vi "Length_15.vi"() -> ()   [LabVIEW 2020]
uses:
  Support/Controls/Cmd_Mouse Popup.ctl
  Support/Controls/Clst_Initialize Input.ctl
  Support/Controls/Clst_Result inspec.ctl
  Support/Controls/Cmd_Var Data IO.ctl
  Variables/Global_Cal Info.vi
panel:
  out "Measured 3":string[][](table) caption="○ 평면도 계산결과 (μm)"
  in  "Measured 2":string[][](table) caption="○ 반복정밀도"
  in  "STD select":string(combo)="1" caption="기준기 Range"
  in  "Spec 변경":bool
  in  "Random":bool
  out "Spec":string[][](table) caption="Spec (명목 직경)"
  out "제목":string
  out "에러 출력":errorcluster
  out "Condition":string[][](table) caption="○ 측정 조건"
  in  "Measured":string[][](table) caption="○ 평면도 측정결과 ( ˝ )"
  out "Load?":bool
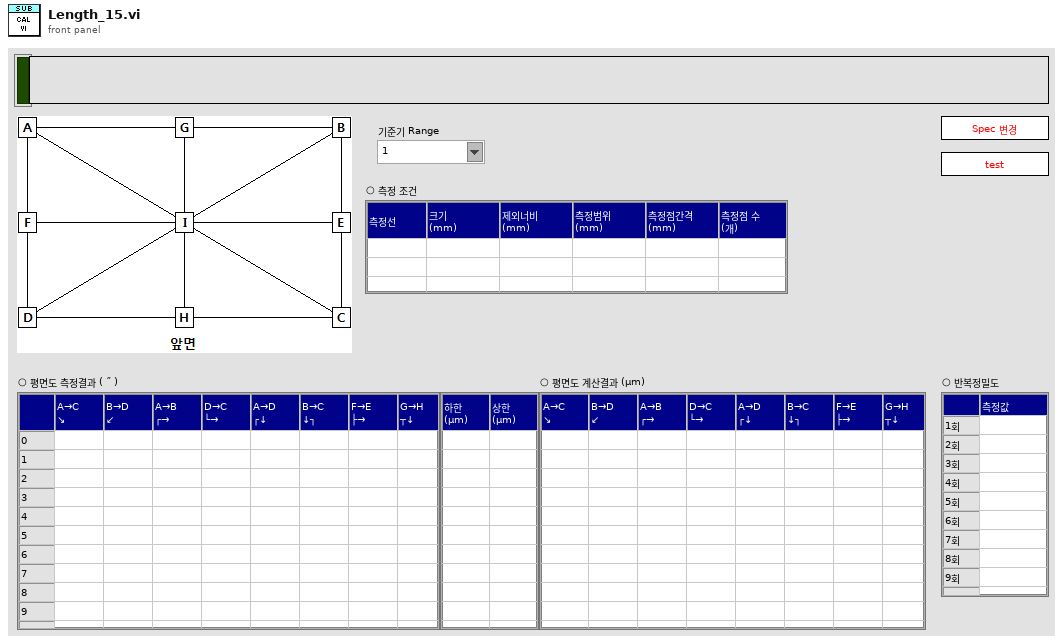
[diagram p1: front panel]
types:
  T1 = typedef "Cmd_Mouse Popup.ctl" = enum16{"활성화", "메뉴선택"}
  T2 = cluster{"Shift":bool, "Ctrl":bool, "Alt":bool, "Cmd":bool, "Opt":bool}
  T3 = typedef "Clst_Initialize Input.ctl" = cluster{"Initialize 1":cluster{"Condition":refnum<vi>[], "Spec":refnum<vi>[], "Measured":refnum<vi>[], "Resolution":refnum<vi>[], "Func_ext":string, "제목":refnum<vi>, "Measured_ADJ":refnum<vi>[]}, "Initialize 2":cluster{"문자열":refnum<vi>[], "콤보박스":refnum<vi>[], "링":refnum<vi>[], "열거형":refnum<vi>[], "테이블":refnum<vi>[], "여러열":refnum<vi>[], "디지털(DBL)":refnum<vi>[], "3D string":refnum<vi>[], "ctrl":refnum<vi>[], "boolean":refnum<vi>[]}}
  T4 = typedef "Clst_Result inspec.ctl" = cluster{"분해능":string, "문자열 1":string, "문자열 2":string, "숫자형 1":i32, "숫자형 2":i32, "숫자형 3":dbl, "문자배열 1D":string[], "문자배열 2D":string[][], "문자배열 3D":string[][][], "문자배열 4D":string[][][][], "불리언 1D":bool[]}
  T5 = typedef "Cmd_Var Data IO.ctl" = enum16{"Condition", "Condition Default", "Condition_Temp", "Resolution", "Resolution Default", "Resolution Old", "Spec", "Spec Default", "Spec Old", "Spec Temp", "Result", "Result2", "Result3", "Result_Temp", "Result_ADJ", "Result_ADJ2", "STD1", "STD2", "STD3", "STD4", "STD5", "STD Temp", "CMC", "CMC Default"}
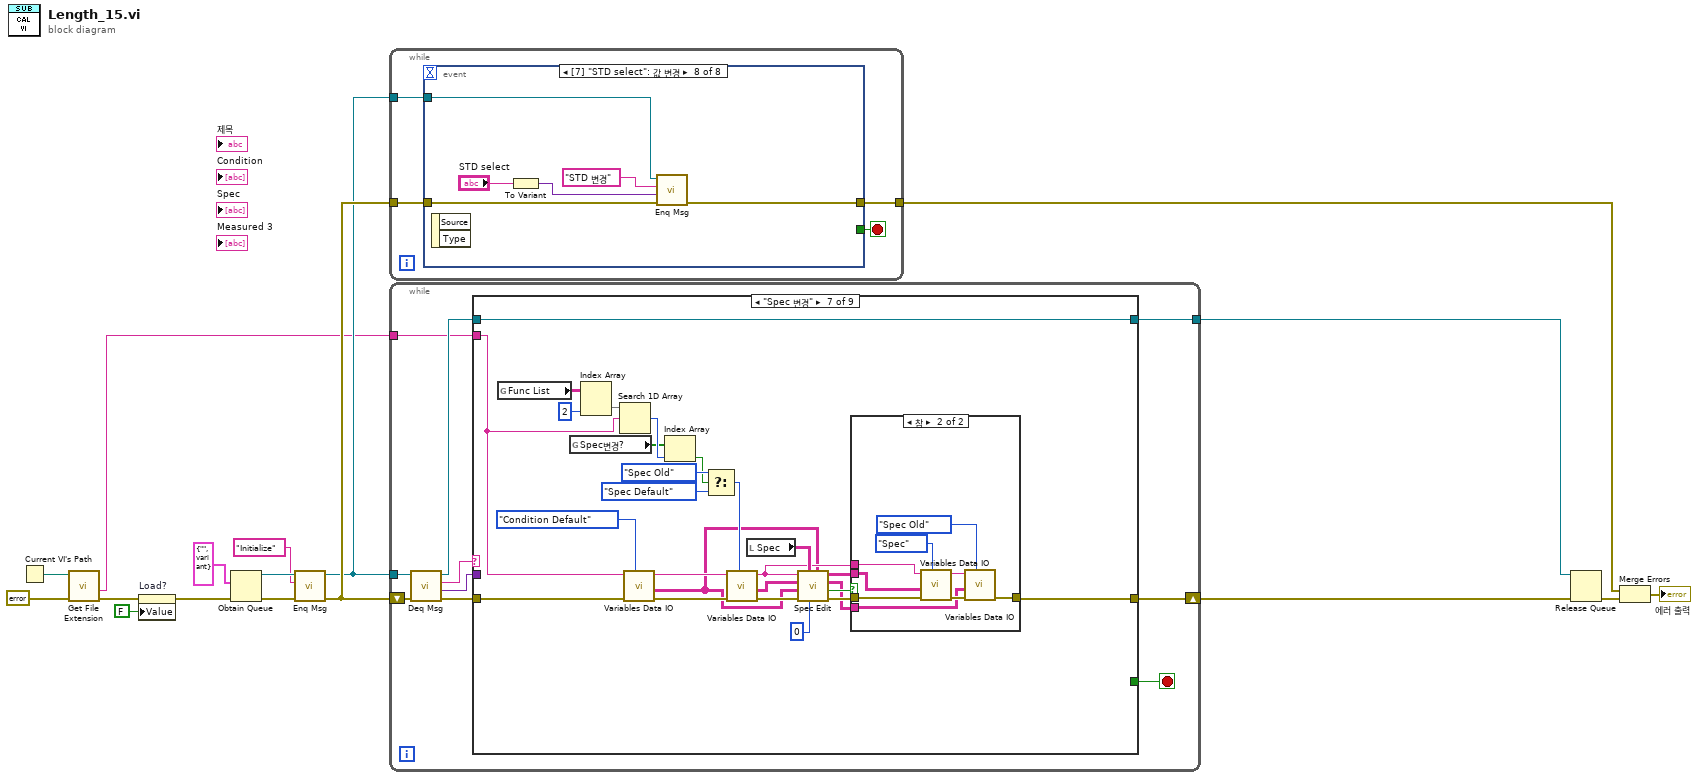
[diagram p0: block diagram]
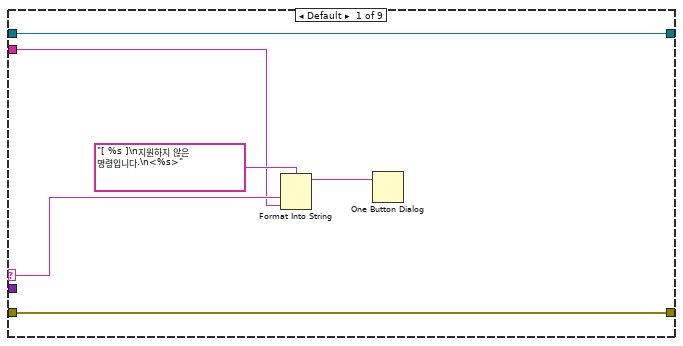
[diagram p2: hidden frame]
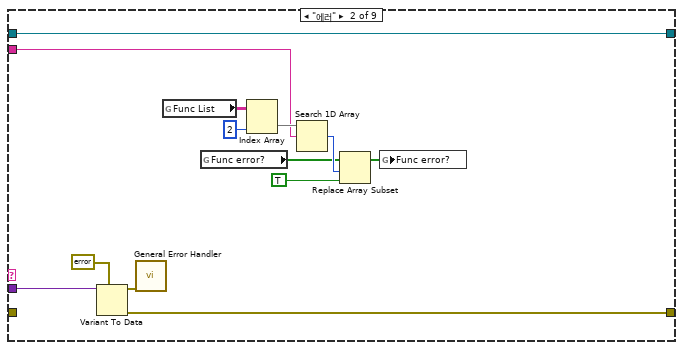
[diagram p3: hidden frame]
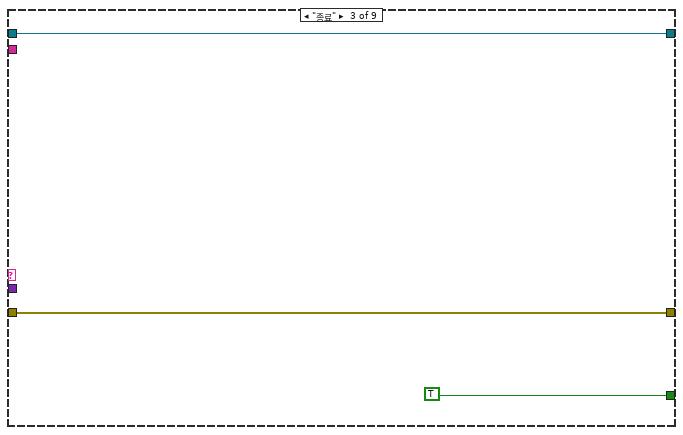
[diagram p4: hidden frame]
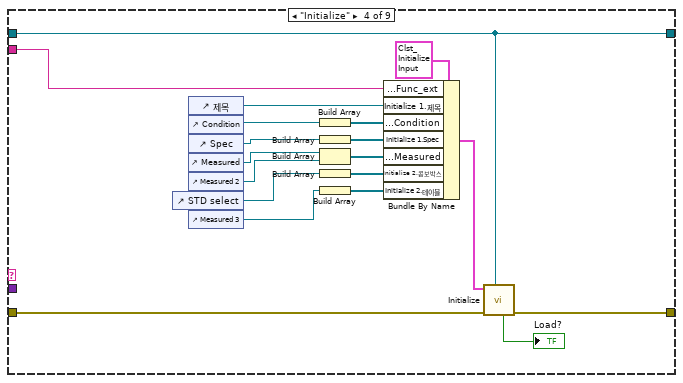
[diagram p5: hidden frame]
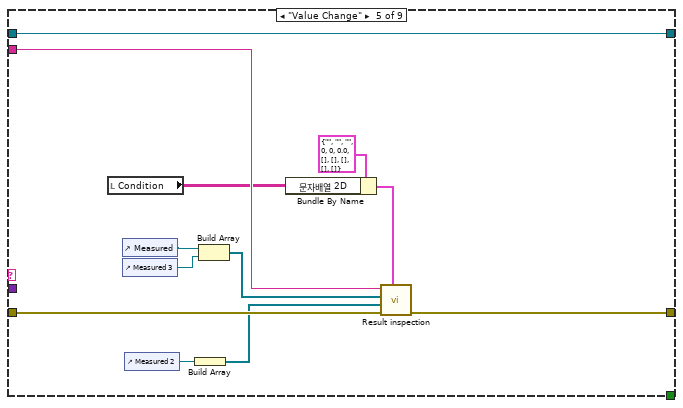
[diagram p6: hidden frame]
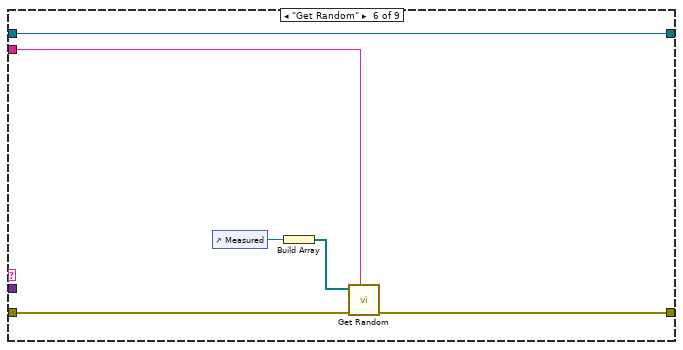
[diagram p7: hidden frame]
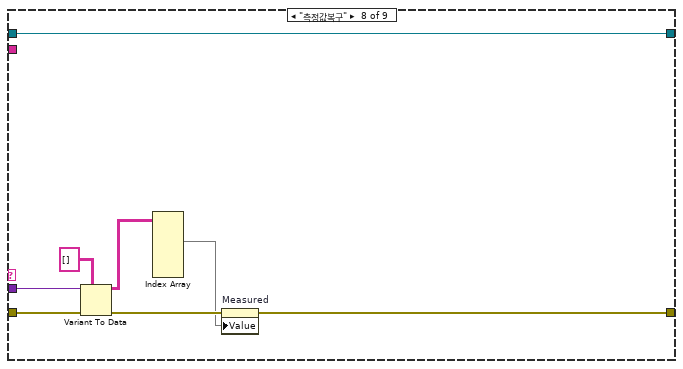
[diagram p9: hidden frame]
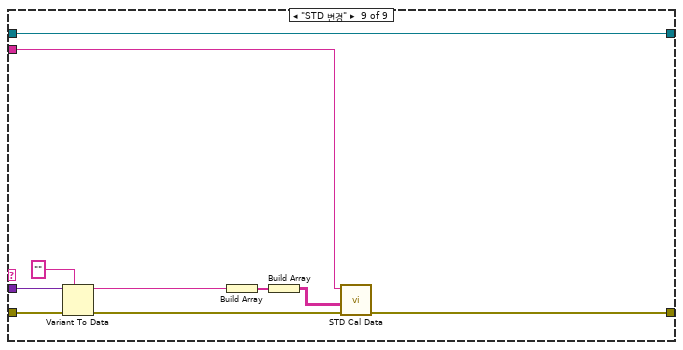
[diagram p10: hidden frame]
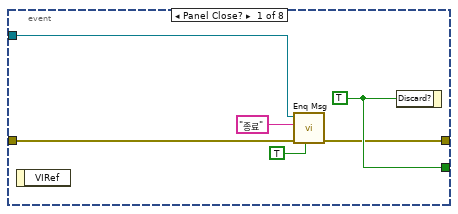
[diagram p11: hidden frame]
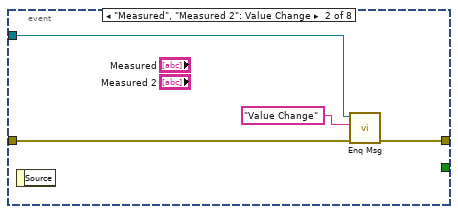
[diagram p12: hidden frame]
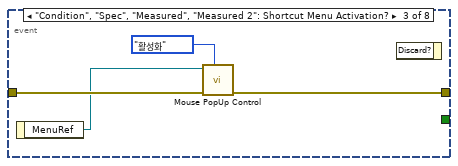
[diagram p13: hidden frame]
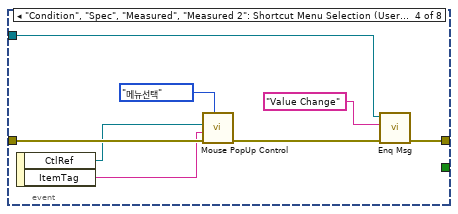
[diagram p14: hidden frame]
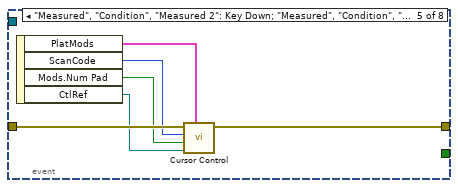
[diagram p15: hidden frame]
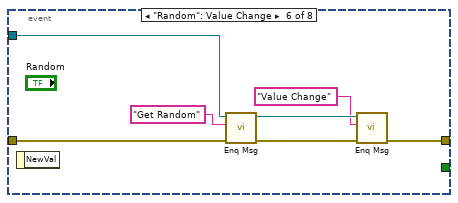
[diagram p16: hidden frame]
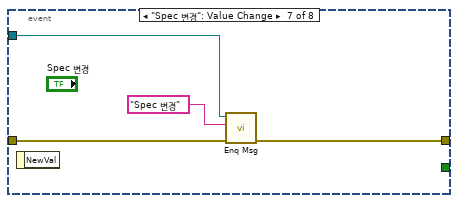
[diagram p17: hidden frame]
diagram:
  n1 = Current VI's Path() -> (path=w5:path)
  n2 = call <vilib>:"Get File Extension.vi"("error in (no error)"=errorcluster {"status"=FALSE, "code"=0, "source"=""} ("에러 상수"), "file"=w5) -> ("error out"=w3:errorcluster, "filename without extension"=w4:string)  [unwired: 5 in, 3 out]
  n3 = property on="Load?" class="Bool (엄격한)"(error in=w3, "Value"=FALSE ("Load?")) -> (error out=w2:errorcluster)  [unwired: 1 in, 1 out]
  n4 = Obtain Queue(element data type=cluster{"메세지":string, "값":variant} {"메세지"="", "값"=variant} ("Message Cluster"), error in (no error)=w2) -> (queue out=w14:refnum<queue>, error out=w16:errorcluster)  [unwired: 3 in, 1 out]
  n5 = call "Enq Msg.vi"("에러 입력(에러 없음)"=w16, "메세지"="Initialize", "큐 입력"=w14) -> ("에러 출력"=w15:errorcluster, "큐 출력"=w12:refnum<queue>)  [unwired: 7 in]
  n6 = while {
    tunnel: w15 -> [w19]
    tunnel: w12 -> [w20]
    tunnel: [w18] -> w9
    stop <- w21 stop-if-true
    n7 = event shown="[7] \"STD select\": 값 변경" {
      selector: _ -> [_ _ _ _ _ _ _ _]
      dyn-events: _ -> [_ _ _ _ _ _ _ _]
      timeout: _ -> [_ _ _ _ _ _ _ _]
      tunnel: [w27 _ _ _ _ _ _ _] -> w21
      tunnel: w20 -> [w25 w31 _ w36 _ w54 w58 w64]
      tunnel: w19 -> [w26 w29 w35 w43 w49 w55 w59 w65]
      tunnel: [w23 w30 w34 w37 w48 w50 w57 w63] -> w18
      event Panel Close? {
        w27 = TRUE ("버림?")
        n8 = event-data() -> ()  [unwired: 1 in, 1 out]
        n9 = call "Enq Msg.vi"("우선순위 메시지?"=TRUE, "에러 입력(에러 없음)"=w26, "메세지"="종료", "큐 입력"=w25) -> ("에러 출력"=w23:errorcluster)  [unwired: 6 in, 1 out]
        n10 = event-data("Discard?"=w27) -> ()  [unwired: 1 in, 1 out]
      }
      event "Measured", "Measured 2": Value Change {
        n11 = event-data() -> ()  [unwired: 1 in, 1 out]
        n12 = call "Enq Msg.vi"("에러 입력(에러 없음)"=w29, "메세지"="Value Change", "큐 입력"=w31) -> ("에러 출력"=w30:errorcluster)  [unwired: 7 in, 1 out]
      }
      event "Condition", "Spec", "Measured", "Measured 2": Shortcut Menu Activation? {
        n13 = event-data() -> ("MenuRef"=w33:refnum<k9>)  [unwired: 1 in]
        n14 = call "Mouse PopUp Control.vi"("type"=Cmd_Mouse_Popup."활성화", "error in"=w35, "메뉴 참조"=w33) -> ("error out"=w34:errorcluster)  [unwired: 8 in]
        n15 = event-data() -> ()  [unwired: 2 in, 1 out]
      }
      event "Condition", "Spec", "Measured", "Measured 2": Shortcut Menu Selection (User) {
        n16 = event-data() -> ("CtlRef"=w41:refnum<vi>, "ItemTag"=w40:string)  [unwired: 1 in]
        n17 = call "Mouse PopUp Control.vi"("type"=Cmd_Mouse_Popup."메뉴선택", "error in"=w43, "아이템 태그"=w40, "Tbl 참조 번호"=w41) -> ("error out"=w38:errorcluster)  [unwired: 7 in]
        n18 = call "Enq Msg.vi"("에러 입력(에러 없음)"=w38, "메세지"="Value Change", "큐 입력"=w36) -> ("에러 출력"=w37:errorcluster)  [unwired: 7 in, 1 out]
      }
      event "Measured", "Condition", "Measured 2": Key Down; "Measured", "Condition", "Measured 2": Key Repeat {
        n19 = event-data() -> ("PlatMods"=w44:T2, "ScanCode"=w47:i16, "Mods.Num Pad"=w46:bool, "CtlRef"=w45:refnum<vi>)  [unwired: 1 in]
        n20 = call "Cursor Control.vi"("플랫폼 조합키"=w44, "참조"=w45, "Num Pad"=w46, "ScanCode"=w47, "error in"=w49) -> ("error out"=w48:errorcluster)  [unwired: 5 in, 1 out]
      }
      event "Random": Value Change {
        n21 = event-data() -> ()  [unwired: 1 in, 1 out]
        n22 = call "Enq Msg.vi"("에러 입력(에러 없음)"=w55, "메세지"="Get Random", "큐 입력"=w54) -> ("에러 출력"=w53:errorcluster, "큐 출력"=w52:refnum<queue>)  [unwired: 7 in]
        n23 = call "Enq Msg.vi"("에러 입력(에러 없음)"=w53, "메세지"="Value Change", "큐 입력"=w52) -> ("에러 출력"=w50:errorcluster)  [unwired: 7 in, 1 out]
      }
      event "Spec 변경": Value Change {
        n24 = event-data() -> ()  [unwired: 1 in, 1 out]
        n25 = call "Enq Msg.vi"("에러 입력(에러 없음)"=w59, "메세지"="Spec 변경", "큐 입력"=w58) -> ("에러 출력"=w57:errorcluster)  [unwired: 7 in, 1 out]
      }
      event "STD select": Value Change {
        n26 = event-data() -> ()  [unwired: 1 in, 2 out]
        n27 = To Variant(anything="STD select") -> (Variant=w61:variant)
        n28 = call "Enq Msg.vi"("에러 입력(에러 없음)"=w65, "값"=w61, "메세지"="STD 변경", "큐 입력"=w64) -> ("에러 출력"=w63:errorcluster)  [unwired: 6 in, 1 out]
      }
    }
  }
  n29 = while {
    shift-right: [w76] -> w11
    shift-left: w15 -> [w75]
    tunnel: w12 -> [w73]
    tunnel: [w68] -> w10
    tunnel: w4 -> [w67]
    stop <- w69 stop-if-true
    n30 = call "Deq Msg.vi"("에러 입력(에러 없음)"=w75, "큐 입력"=w73) -> ("에러 출력"=w74:errorcluster, "값"=w70:variant, "메세지"=w72:string, "큐 출력"=w71:refnum<queue>)  [unwired: 6 in]
    n31 = case shown="\"Spec 변경\"" w72 {
      selector: w72 -> [w78 _ _ _ _ _ _ _ _]
      tunnel: w74 -> [w82 _ w98 w117 w124 w131 w155 w176 w188]
      tunnel: [w82 w92 w98 w106 w128 w132 w157 w172 w184] -> w76
      tunnel: w71 -> [w81 w91 w96 w105 w129 w135 w161 w179 w189]
      tunnel: w70 -> [_ w93 _ _ _ _ _ w177 w187]
      tunnel: [_ _ TRUE ("버림?") _ _ _ _ _ _] -> w69
      tunnel: [w81 w91 w96 w105 w129 w135 w161 w179 w189] -> w68
      tunnel: w67 -> [w77 w83 _ w107 w127 w130 w141 _ w180]
      frame Default {
        n32 = Format Into String(format string="[ %s ]\n지원하지 않은 명령입니다.\n<%s>" ("메시지"), w78, w77) -> (resulting string=w79:string)  [unwired: 2 in, 1 out]
        n33 = One Button Dialog(message=w79) -> ()  [unwired: 1 in, 1 out]
      }
      frame "에러" {
        n34 = Variant To Data(type=errorcluster {"status"=FALSE, "code"=0, "source"=""} ("에러 출력"), Variant=w93) -> (data=w95:errorcluster, error out=w92:errorcluster)  [unwired: 1 in]
        n35 = call <vilib>:"General Error Handler.vi"("error in (no error)"=w95) -> ()  [unwired: 10 in, 5 out]
        n36 = global read "Global_Cal Info.vi" "Func List"() -> (w85:string[][])
        n37 = global read "Global_Cal Info.vi" "Func error?"() -> (w88:bool[])
        n38 = Index Array(array=w85, index (col)=2 ("비활성화된 인덱스 (열)")) -> (element=w86:string[])  [unwired: 1 in]
        n39 = Search 1D Array(1D array=w86, element=w83) -> (index of element=w89:i32)  [unwired: 1 in]
        n40 = Replace Array Subset(array=w88, new element=TRUE ("새 원소/부분배열"), index=w89) -> (w90:bool[])
        n41 = global write "Global_Cal Info.vi" "Func error?"(w90) -> ()
      }
      frame "종료" {
      }
      frame "Initialize" {
        n42 = control-ref of="STD select"() -> (w103:refnum<vi>)
        n43 = control-ref of="제목"() -> (w110:refnum<vi>)
        n44 = control-ref of="Condition"() -> (w114:refnum<vi>)
        n45 = control-ref of="Spec"() -> (w109:refnum<vi>)
        n46 = control-ref of="Measured"() -> (w111:refnum<vi>)
        n47 = control-ref of="Measured 2"() -> (w101:refnum<vi>)
        n48 = control-ref of="Measured 3"() -> (w100:refnum<vi>)
        n49 = Build Array(w114) -> (w113:refnum<vi>[])
        n50 = Build Array(w109) -> (w108:refnum<vi>[])
        n51 = Build Array(w111, w101) -> (w112:refnum<vi>[])
        n52 = Build Array(w103) -> (w102:refnum<vi>[])
        n53 = Build Array(w100) -> (w99:refnum<vi>[])
        n54 = Bundle By Name(cluster=T3 {"Initialize 1"={"Condition"=[], "Spec"=[], "Measured"=[], "Resolution"=[], "Func_ext"="", "제목"=refnum, "Measured_ADJ"=[]}, "Initialize 2"={"문자열"=[], "콤보박스"=[], "링"=[], "열거형"=[], "테이블"=[], "여러열"=[], "디지털(DBL)"=[], "3D string"=[], "ctrl"=[], "boolean"=[]}} ("입력 클러스터"), "Initialize 1.Func_ext"=w107, "Initialize 1.제목"=w110, "Initialize 1.Condition"=w113, "Initialize 1.Spec"=w108, "Initialize 1.Measured"=w112, "Initialize 2.콤보박스"=w102, "Initialize 2.테이블"=w99) -> (w115:T3)
        n55 = call "Initialize.vi"("큐 입력"=w105, "error in"=w117, "입력 클러스터"=w115) -> ("error out"=w106:errorcluster, "Load?"=→"Load?":bool)  [unwired: 5 in, 2 out]
      }
      frame "Value Change" {
        n56 = local read "Condition"() -> (w119:string[][])
        n57 = control-ref of="Measured"() -> (w126:refnum<vi>)
        n58 = control-ref of="Measured 3"() -> (w123:refnum<vi>)
        n59 = control-ref of="Measured 2"() -> (w122:refnum<vi>)
        n60 = Build Array(w122) -> (w121:refnum<vi>[])
        n61 = Build Array(w126, w123) -> (w125:refnum<vi>[])
        n62 = Bundle By Name(cluster=T4 {"분해능"="", "문자열 1"="", "문자열 2"="", "숫자형 1"=0, "숫자형 2"=0, "숫자형 3"=0.0, "문자배열 1D"=[], "문자배열 2D"=[], "문자배열 3D"=[], "문자배열 4D"=[], "불리언 1D"=[]} ("입력 클러스터"), "문자배열 2D"=w119) -> (w118:T4)
        n63 = call "Result inspection.vi"("입력 클러스터"=w118, "error in"=w124, "Ref. Data (excluded)"=w121, "Ref. Data (Inspection)"=w125, "Func ext"=w127) -> ("error out"=w128:errorcluster)  [unwired: 3 in, 3 out]
      }
      frame "Get Random" {
        n64 = control-ref of="Measured"() -> (w134:refnum<vi>)
        n65 = Build Array(w134) -> (w133:refnum<vi>[])
        n66 = call "Get Random.vi"("Func_Ext"=w130, "에러 입력"=w131, "Meas"=w133) -> ("에러 출력"=w132:errorcluster)  [unwired: 7 in, 1 out]
      }
      frame "Spec 변경" {
        n67 = global read "Global_Cal Info.vi" "Func List"() -> (w146:string[][])
        n68 = global read "Global_Cal Info.vi" "Spec변경?"() -> (w142:bool[])
        n69 = Index Array(array=w146, index (col)=2 ("비활성화된 인덱스 (열)")) -> (element=w144:string[])  [unwired: 1 in]
        n70 = Search 1D Array(1D array=w144, element=w141) -> (index of element=w143:i32)  [unwired: 1 in]
        n71 = call "Variables Data IO.vi"("Select"=Cmd_Var_Data_IO."Condition Default", "error in"=w155, "Func_ext"=w141) -> ("error out"=w139:errorcluster, "Data Out"=w136:string[][], "Func_ext Out"=w138:string)  [unwired: 6 in]
        n72 = Index Array(array=w142, index=w143) -> (element=w147:bool)
        n73 = Select(t=Cmd_Var_Data_IO."Spec Old" ("Select"), s=w147, f=Cmd_Var_Data_IO."Spec Default" ("Select")) -> (s? t:f=w140:T5)
        n74 = call "Variables Data IO.vi"("Select"=w140, "error in"=w139, "Func_ext"=w138) -> ("error out"=w156:errorcluster, "Data Out"=w150:string[][], "Func_ext Out"=w151:string)  [unwired: 6 in]
        n75 = local read "Spec"() -> (w152:string[][])
        n76 = call "Spec Edit.vi"("Condition"=w136, "열번호(기준값)"=0, "Spec Value"=w152, "에러 입력(에러 없음)"=w156, "Resolution"=w136, "Spec Default"=w150, "Func_ext"=w151) -> ("에러 출력"=w158:errorcluster, "변경?"=w159:bool, "Spec Default out"=w154:string[][], "Spec 출력"=w160:string[][])  [unwired: 1 in]
        n77 = case shown="참" w159 {
          tunnel: w160 -> [_ w163]
          tunnel: w158 -> [w162 w171]
          tunnel: [w162 w167] -> w157
          tunnel: w151 -> [_ w169]
          tunnel: w154 -> [_ w165]
          frame False {
          }
          frame True {
            n78 = call "Variables Data IO.vi"("Select"=Cmd_Var_Data_IO."Spec", "error in"=w171, "Data In"=w163, "Func_ext"=w169) -> ("error out"=w168:errorcluster, "Func_ext Out"=w166:string)  [unwired: 5 in, 1 out]
            n79 = call "Variables Data IO.vi"("Select"=Cmd_Var_Data_IO."Spec Old", "error in"=w168, "Data In"=w165, "Func_ext"=w166) -> ("error out"=w167:errorcluster)  [unwired: 5 in, 2 out]
          }
        }
      }
      frame "측정값복구" {
        n80 = Variant To Data(error in=w176, type=string[][][] [], Variant=w177) -> (data=w174:string[][][], error out=w175:errorcluster)
        n81 = Index Array(array=w174) -> (element #1=w173:string[][])  [unwired: 6 in, 1 out]
        n82 = property on="Measured" class="Tbl (엄격한)"(error in=w175, "Value"=w173) -> (error out=w172:errorcluster)  [unwired: 1 in, 1 out]
      }
      frame "STD 변경" {
        n83 = Variant To Data(error in=w188, type="", Variant=w187) -> (data=w183:string, error out=w185:errorcluster)
        n84 = Build Array(w183) -> (w182:string[])
        n85 = Build Array(w182) -> (w181:string[][])
        n86 = call "STD Cal Data.vi"("error in"=w185, "Data in"=w181, "Func_ext"=w180) -> ("error out"=w184:errorcluster)  [unwired: 4 in, 4 out]
      }
    }
  }
  n87 = Release Queue(queue=w10, error in (no error)=w11) -> (error out=w8:errorcluster)  [unwired: 1 in, 2 out]
  n88 = Merge Errors(w9, w8) -> (→"에러 출력":errorcluster)
